vi "Teleop Shooter Control.vi"(8 "D-Pad Down Pressed?":bool, 9 "D-Pad Up Pressed?":bool, 11 "Joystick Value":dbl) -> (2 "D-Pad Output":dbl, 3 "Joystick Output":dbl)   [LabVIEW 2016]
uses:
  <vilib>/ptbypt/NI_PtbyPt.lvlib
panel:
  in  "D-Pad Control":dbl=0.05
  in  "Joystick Multiplier":dbl=0.1
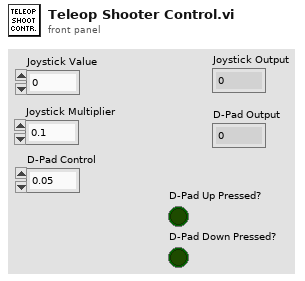
[diagram p1: front panel]
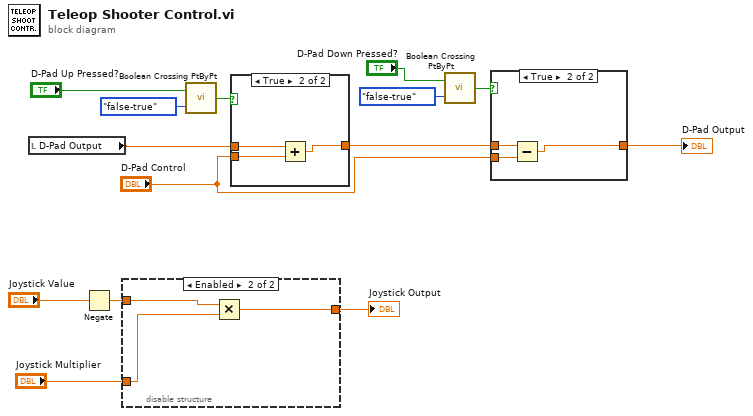
[diagram p0: block diagram]
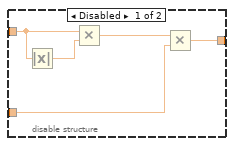
[diagram p2: hidden frame]
diagram:
  n1 = local read "D-Pad Output"() -> (w1:dbl)
  n2 = Negate(x="Joystick Value") -> (-x=w14:dbl)
  n3 = disable-structure shown="Enabled" {
    disable-tunnel: w14 -> [w18 w22]
    disable-tunnel: "Joystick Multiplier" -> [w16 w21]
    disable-tunnel: [w15 w20] -> w11
    frame Disabled {
      n4 = Absolute Value(x=w18) -> (abs(x)=w19:dbl)
      n5 = Multiply(x=w18, y=w19) -> (x*y=w17:dbl)
      n6 = Multiply(x=w17, y=w16) -> (x*y=w15:dbl)
    }
    frame Enabled {
      n7 = Multiply(x=w22, y=w21) -> (x*y=w20:dbl)
    }
  }
  "Joystick Output" <- w11
  n8 = call <vilib>:"Boolean Crossing PtByPt.vi"("direction"=enum16{"either", "false-true", "true-false"}."false-true", "input"="D-Pad Up Pressed?") -> ("crossing"=w8:bool)  [unwired: 1 in]
  n9 = case shown="True" w8 {
    tunnel: w1 -> [w23 w26]
    tunnel: "D-Pad Control" -> [_ w25]
    tunnel: [w23 w24] -> w4
    frame False {
    }
    frame True {
      n10 = Add(x=w26, y=w25) -> (x+y=w24:dbl)
    }
  }
  n11 = call <vilib>:"Boolean Crossing PtByPt.vi"("direction"=enum16{"either", "false-true", "true-false"}."false-true", "input"="D-Pad Down Pressed?") -> ("crossing"=w6:bool)  [unwired: 1 in]
  n12 = case shown="True" w6 {
    tunnel: w4 -> [w27 w29]
    tunnel: "D-Pad Control" -> [_ w30]
    tunnel: [w27 w28] -> w2
    frame False {
    }
    frame True {
      n13 = Subtract(x=w29, y=w30) -> (x-y=w28:dbl)
    }
  }
  "D-Pad Output" <- w2
